vi "Reset.vi"(8 "error in (no error)":errorcluster, 11 "2230G in":refnum<class "2230G.lvclass">) -> (0 "error out":errorcluster, 3 "2230G out":refnum<class "2230G.lvclass">)   [LabVIEW 2018, in "2230G.lvlib" / "2230G.lvclass"]
uses:
  2230G.lvclass
  PPLs/Power Supply/Parent/Power_Supply.lvlibp/Power Supply.lvclass
  <instrlib>/Keithley KE22xx Series/Keithley KE22xx Series.lvlib
  C:/Projects/LabVIEW/PPLs/Power Supply/Parent/Power_Supply.lvlibp/Power Supply.lvclass
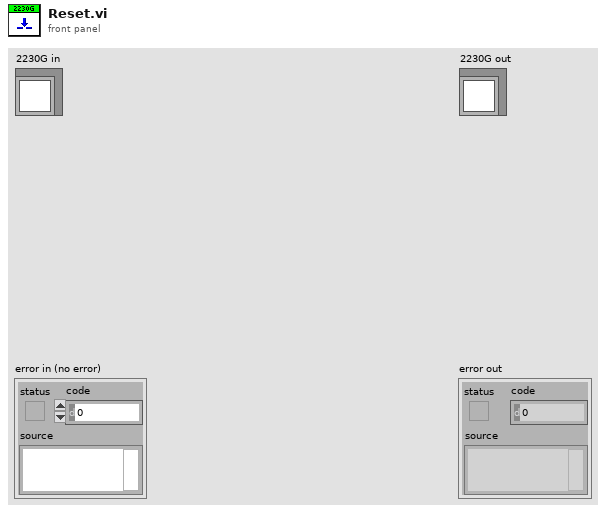
[diagram p1: front panel]
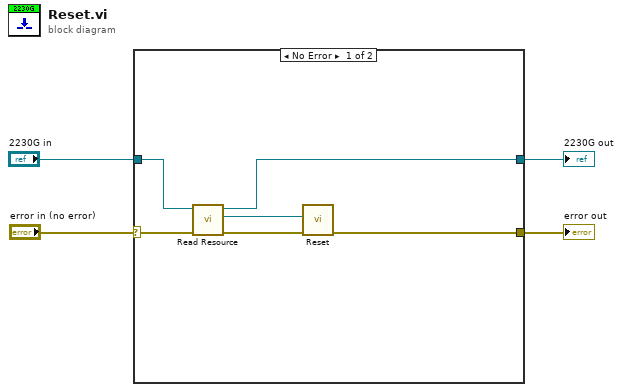
[diagram p0: block diagram]
diagram:
  n1 = case shown="No Error" "error in (no error)" {
    selector: "error in (no error)" -> [w10 w12]
    tunnel: [w5 w12] -> w3
    tunnel: [w6 w11] -> w2
    tunnel: "2230G in" -> [w9 w11]
    frame No Error {
      n2 = call "Read Resource.vi"("error in"=w10, "Power Supply in"=w9) -> ("error out"=w8:errorcluster, "Resource"=w7:refnum<visa-resource-name>, "Power Supply out"=w6:refnum<class "2230G.lvclass">)  [unwired: 7 in]
      n3 = call <instrlib>:"Reset.vi"("error in (no error)"=w8, "VISA resource name"=w7) -> ("error out"=w5:errorcluster)  [unwired: 8 in, 1 out]
    }
    frame Error {
    }
  }
  "error out" <- w3
  "2230G out" <- w2
